vi "DangerousToy.vi"() -> ()   [LabVIEW 2018]
uses:
  <vilib>/Analysis/baseanly.llb/Mean (DBL).vi
  <vilib>/Analysis/NI_AAL_SigProc.lvlib
  <vilib>/Analysis/NI_AALBase.lvlib
panel:
  out "Signals 2":dbl[](graph) caption="Signals"
  out "omega":dbl
  out "damping rate (alpha)":dbl
  out "total amplitude decline \nrate over 10 iteration\n(damping rate)":dbl
  out "width":dbl
  out "number of samples":dbl
  out "half period":dbl
  out "frequency":dbl
  out "T (period)":dbl
  out "total value of T \nin 10 iteration":dbl
  in  "width":i32=3 min=3
  out "# found":i32
  out "amplitude":dbl[](array[numeric])
  out "Peak Locations (n)":dbl[](array[numeric])
  out "Signals":dynamicdata(graph)
  out "File Directory":path
  # "67"
  # "10x less"
  # "f = 1/T"
  # "w = 2pi(f)"
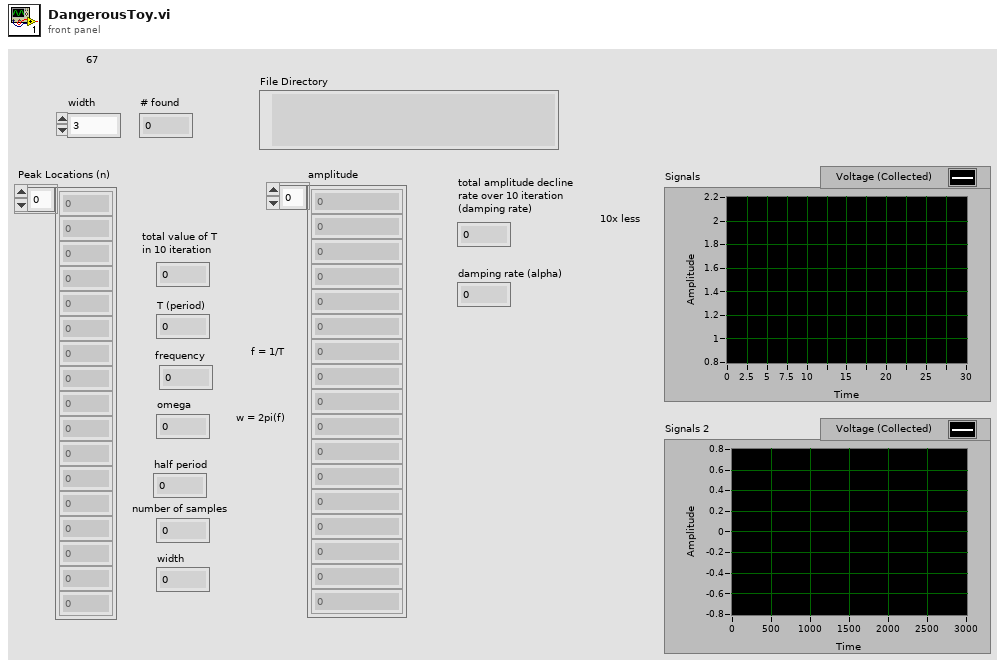
[diagram p1: front panel]
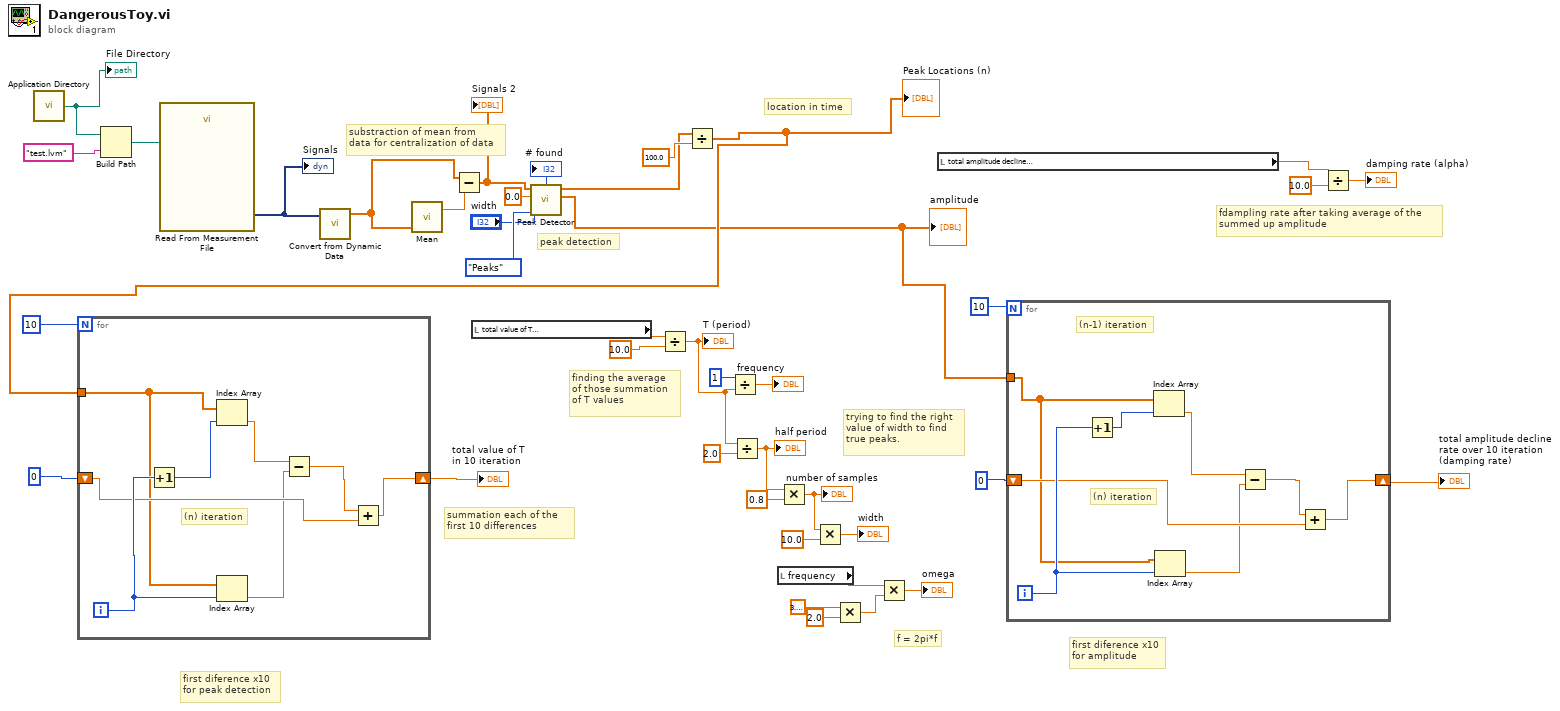
[diagram p0: block diagram]
diagram:
  # "trying to find the right\nvalue of width to find\ntrue peaks."
  # "peak detection"
  # "substraction of mean from\ndata for centralization of data"
  # "fdampling rate after taking average of the \nsummed up amplitude"
  # "first diference x10\nfor amplitude"
  # "f = 2pi*f"
  # "finding the average\nof those summation\nof T values"
  # "summation each of the \nfirst 10 differences"
  # "first diference x10\nfor peak detection"
  # "location in time"
  n1 = call <vilib>:"Application Directory.vi"() -> ("Application Directory"=w40:path)
  "File Directory" <- w40
  n2 = Build Path(base path=w40, name or relative path="test.lvm") -> (appended path=w38:path)
  n3 = call "Read From Measurement File"("Filename"=w38) -> ("Signals"=w30:dynamicdata)  [unwired: 5 in, 5 out]
  "Signals" <- w30
  n4 = call "Convert from Dynamic Data"("Dynamic Data Type"=w30) -> ("Array"=w31:dbl[])  [unwired: 3 in]
  n5 = call-poly <vilib>:"Mean.vi"("X"=w31) -> ("mean"=w32:dbl)  [unwired: 1 out]
  n6 = Subtract(x=w31, y=w32) -> (x-y=w1:dbl[])
  "Signals 2" <- w1
  n7 = local read "total value of T \nin 10 iteration"() -> (w27:dbl)
  n8 = call <vilib>:"Peak Detector.vi"("peaks/valleys"=enum32{"Peaks", "Valleys"}."Peaks", "width"="width", "threshold"=0.0, "X"=w1) -> ("Amplitudes"=w3:dbl[], "Locations"=w2:dbl[], "# found"=→"# found":i32)  [unwired: 3 in, 2 out]
  "amplitude" <- w3
  n9 = Divide(x=w27, y=10.0) -> (x/y=w20:dbl)
  "T (period)" <- w20
  n10 = Divide(x=w2, y=100.0) -> (x/y=w4:dbl[])
  "Peak Locations (n)" <- w4
  n11 = for {
    N: 10 -> [_]
    shift-right: [w41] -> w28
    shift-left: 0 -> [w45]
    tunnel: w4 -> [w43]
    i -> [w46]
    # "(n) iteration"
    n12 = Increment(x=w46) -> (x+1=w47:i32)
    n13 = Index Array(array=w43, index=w47) -> (element=w48:dbl)
    n14 = Index Array(array=w43, index=w46) -> (element=w42:dbl)
    n15 = Subtract(x=w48, y=w42) -> (x-y=w44:dbl)
    n16 = Add(x=w44, y=w45) -> (x+y=w41:dbl)
  }
  "total value of T \nin 10 iteration" <- w28
  n17 = Divide(x=1, y=w20) -> (x/y=→"frequency":dbl)
  n18 = Divide(x=w20, y=2.0) -> (x/y=w22:dbl)
  "half period" <- w22
  n19 = local read "frequency"() -> (w10:dbl)
  n20 = Multiply(x=w22, y=0.8) -> (x*y=w19:dbl)
  "number of samples" <- w19
  n21 = Multiply(x=w19, y=10.0) -> (x*y=→"width":dbl)
  n22 = Multiply(x=3.141592653589793, y=2.0) -> (x*y=w7:dbl)
  n23 = Multiply(x=w10, y=w7) -> (x*y=→"omega":dbl)
  n24 = local read "total amplitude decline \nrate over 10 iteration\n(damping rate)"() -> (w13:dbl)
  n25 = for {
    N: 10 -> [_]
    shift-right: [w53] -> w14
    shift-left: 0 -> [w52]
    tunnel: w3 -> [w51]
    i -> [w55]
    # "(n) iteration"
    # "(n-1) iteration"
    n26 = Increment(x=w55) -> (x+1=w56:i32)
    n27 = Index Array(array=w51, index=w56) -> (element=w50:dbl)
    n28 = Index Array(array=w51, index=w55) -> (element=w49:dbl)
    n29 = Subtract(x=w50, y=w49) -> (x-y=w54:dbl)
    n30 = Add(x=w54, y=w52) -> (x+y=w53:dbl)
  }
  "total amplitude decline \nrate over 10 iteration\n(damping rate)" <- w14
  n31 = Divide(x=w13, y=10.0) -> (x/y=→"damping rate (alpha)":dbl)
